vi "Sample_Finite_DigitalTrigger.vi"() -> ()   [LabVIEW 2013]
doc: "This samples demonstrates how to sample a finite waveform."
uses:
  <userlib>/ArtScope/Trigger/ArtScope_ConfigureTriggerDigital.vi
  <userlib>/ArtScope/Fetch/ArtScope_FetchBinary16.vi
  <userlib>/ArtScope/_SubVI/ArtScope_ArrayByChannel_U16.vi
panel:
  out "error out":errorcluster
  in  "reference position":dbl
  in  "source":string(combo)="VAL_TRIGGER_DTR"
  in  "edge":i32(ring) items=["Negative", "Positive", "NegatPosit"]
  in  "sensitive":i32=50
  in  "count":i32=1
  in  "range(Vpp)":i32(ring) items=["20V", "10V", "2V", "40V", "16V", "8V", "4V", "1.6V", "800m", "400m", "160m", "80m", "40m"]
  in  "offset(mV)":i32
  in  "NumSamples":i32=1000
  in  "Stop":bool
  out "waveform":u16[][](graph)
  in  "Timeout(s)":dbl=10.0
  in  "MinRecordLength":i32=6000
  in  "MinSampleRate":dbl=800000.0
  in  "Coupling":i32(ring) items=["DC", "AC"]
  in  "Channel Name":string="0"
  in  "Resource Name":string="Dev1"
  # "Vertical"
  # "Horizontal"
  # "Trigger"
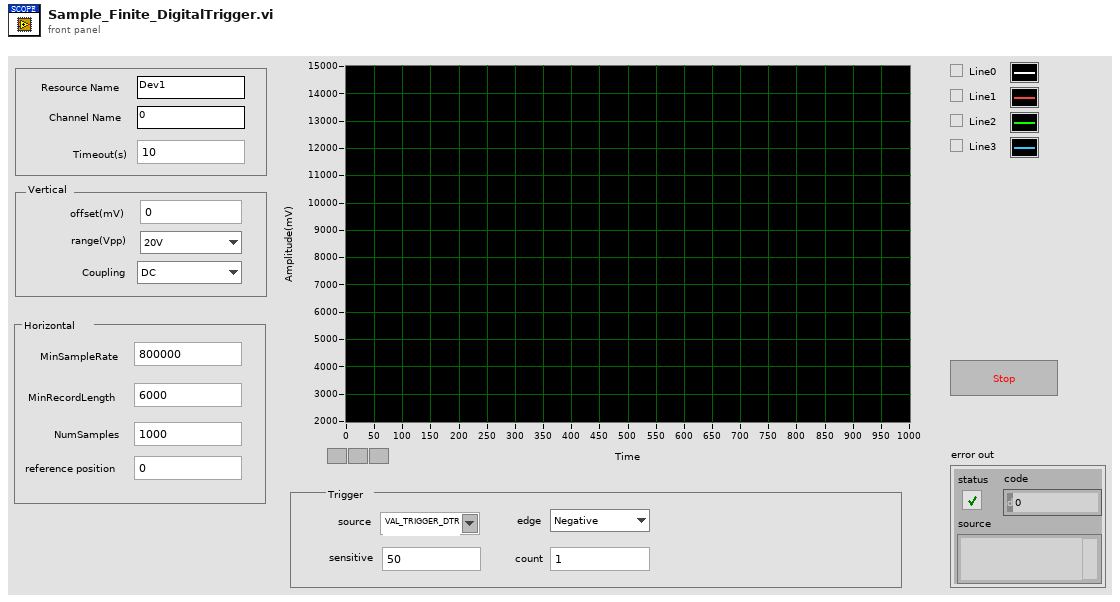
[diagram p1: front panel]
types:
  T1 = cluster{"fLSB":cluster{dbl, dbl, dbl, dbl, dbl, dbl, dbl, dbl}, "RangeValue":cluster{dbl, dbl, dbl, dbl, dbl, dbl, dbl, dbl}, "wMaxLSB":u32, "TriggerMode":i32, "sampLengthPerChan":u32, "pAvailSampsPoints":u32, "channelCount":i32}
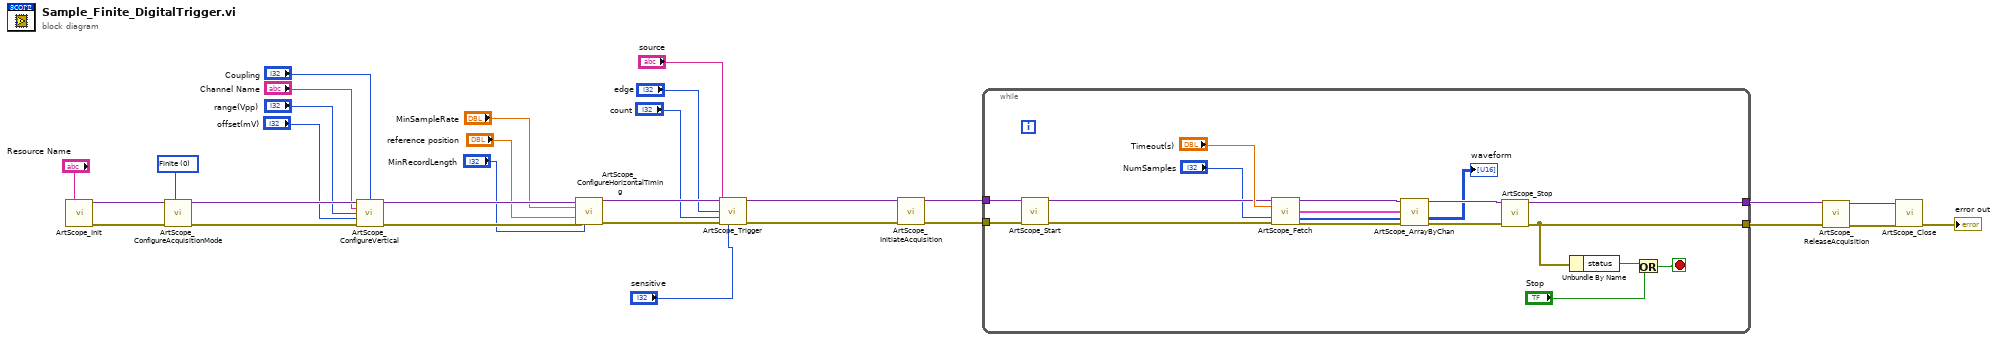
[diagram p0: block diagram]
diagram:
  w23 = 0 items=["Finite", "Continuous"] ("AcuqMode")
  n1 = call <userlib>:"ArtScope_Init.vi"("task name"="Resource Name") -> ("task handle"=w24:variant, "error out"=w25:errorcluster)  [unwired: 13 in]
  n2 = call <userlib>:"ArtScope_ConfigureAcquisitionMode.vi"("task handle"=w24, "acquisition mode"=w23, "error in (no error)"=w25) -> ("task handle"=w22:variant, "error out"=w26:errorcluster)  [unwired: 11 in]
  n3 = call <userlib>:"ArtScope_ConfigureVertical.vi"("task handle"=w22, "coupling"="Coupling", "channels"="Channel Name", "range(Vpp)"="range(Vpp)", "offset"="offset(mV)", "error in (no error)"=w26) -> ("task handle"=w28:variant, "error out"=w27:errorcluster)  [unwired: 8 in]
  n4 = call <userlib>:"ArtScope_ConfigureHorizontalTiming.vi"("task handle"=w28, "min sample rate"="MinSampleRate", "reference position"="reference position", "error in (no error)"=w27, "min record length"="MinRecordLength") -> ("task handle"=w20:variant, "error out"=w21:errorcluster)  [unwired: 9 in]
  n5 = call-poly <userlib>:"ArtScope_Trigger.vi"("task handle"=w20, "trigger source"="source", "edge"="edge", "trigger count"="count", "error in (no error)"=w21, "trigger sensitive"="sensitive") -> ("task handle"=w12:variant, "error out"=w11:errorcluster)  [unwired: 8 in]
  n6 = call <userlib>:"ArtScope_InitiateAcquisition.vi"("task handle"=w12, "error in (no error)"=w11) -> ("task handle"=w10:variant, "error out"=w9:errorcluster)  [unwired: 12 in]
  n7 = while {
    tunnel: [w44] -> w16
    tunnel: [w43] -> w15
    tunnel: w10 -> [w42]
    tunnel: w9 -> [w47]
    stop <- w45 stop-if-true
    n8 = call <userlib>:"ArtScope_Start.vi"("task handle"=w42, "error in (no error)"=w47) -> ("task handle"=w40:variant, "error out"=w39:errorcluster)  [unwired: 12 in]
    n9 = call-poly <userlib>:"ArtScope_Fetch.vi"("task handle"=w40, "timeout"="Timeout(s)", "num samples"="NumSamples", "error in (no error)"=w39) -> ("task handle"=w37:variant, "wfm info"=w33:T1, "data"=w32:u16[], "error out"=w34:errorcluster)  [unwired: 8 in]
    n10 = call-poly <userlib>:"ArtScope_ArrayByChan.vi"("task handle"=w37, "wfm info"=w33, "1D data"=w32, "error in (no error)"=w34) -> ("task handle"=w36:variant, "2D data"=→"waveform":u16[][], "error out"=w35:errorcluster)  [unwired: 9 in]
    n11 = call <userlib>:"ArtScope_Stop.vi"("task handle"=w36, "error in (no error)"=w35) -> ("task handle"=w44:variant, "error out"=w43:errorcluster)  [unwired: 12 in]
    n12 = Unbundle By Name(w43) -> ("status"=w46:bool)
    n13 = Or(x=w46, y="Stop") -> (x .or. y?=w45:bool)
  }
  n14 = call <userlib>:"ArtScope_ReleaseAcquisition.vi"("task handle"=w16, "error in (no error)"=w15) -> ("task handle"=w14:variant, "error out"=w13:errorcluster)  [unwired: 12 in]
  n15 = call <userlib>:"ArtScope_Close.vi"("task handle"=w14, "error in (no error)"=w13) -> ("error out"=→"error out":errorcluster)  [unwired: 13 in]
